vi "Save Acoustic Data.vi"(0 "ID":i32, 1 "base path":path, 5 "Air Temperature":dbl, 7 "Angle":dbl, 9 "Height":dbl, 11 "error in (no error)":errorcluster, 12 "Captured Data":waveform(dbl)) -> (15 "error out":errorcluster)   [LabVIEW 2021]
uses:
  <vilib>/Utility/file.llb/Write Delimited Spreadsheet (DBL).vi
  <vilib>/Utility/file.llb/Write Delimited Spreadsheet (string).vi
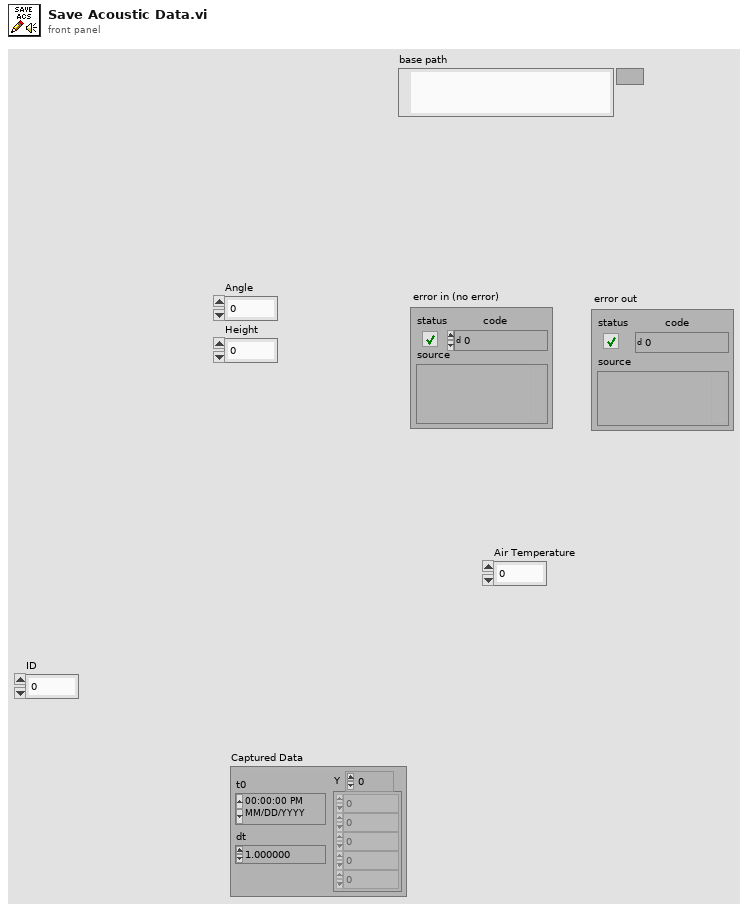
[diagram p1: front panel]
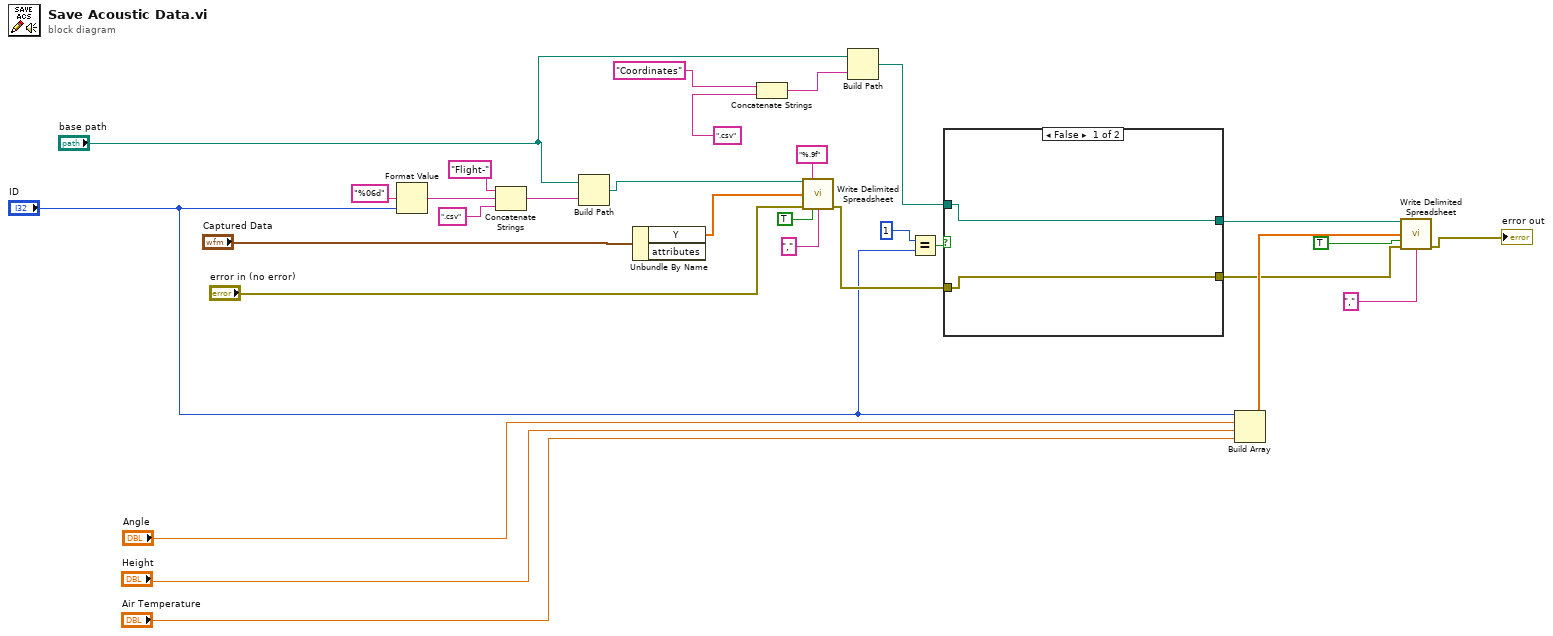
[diagram p0: block diagram]
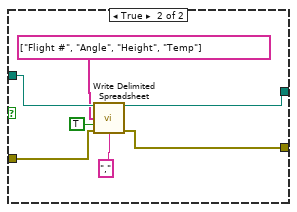
[diagram p2: hidden frame]
diagram:
  n1 = Format Value(format string="%06d", value (0)="ID") -> (output string=w25:string)  [unwired: 1 in]
  n2 = Concatenate Strings("Flight-" ("string"), w25, ".csv") -> (w28:string)
  n3 = Build Path(base path="base path", name or relative path=w28) -> (appended path=w22:path)
  n4 = Unbundle By Name("Captured Data") -> ("Y"=w23:dbl[])  [unwired: 1 out]
  n5 = Concatenate Strings("Coordinates" ("string"), ".csv") -> (w17:string)
  n6 = call-poly <vilib>:"Write Delimited Spreadsheet.vi"("file path (dialog if empty)"=w22, "format (%.3f)"="%.9f" ("format string"), "1D data"=w23, "error in (no error)"="error in (no error)", "transpose? (no:F)"=TRUE, "delimiter (\\t)"="," ("delimiter (Tab)")) -> ("error out"=w4:errorcluster)  [unwired: 8 in, 1 out]
  n7 = Build Path(base path="base path", name or relative path=w17) -> (appended path=w10:path)
  n8 = Equal?(x=1 ("y"), y="ID") -> (x = y?=w11:bool)
  n9 = case shown="False" w11 {
    tunnel: w10 -> [w32 w39]
    tunnel: [w32 w35] -> w6
    tunnel: w4 -> [w31 w34]
    tunnel: [w31 w33] -> w3
    frame False {
    }
    frame True {
      n10 = call-poly <vilib>:"Write Delimited Spreadsheet.vi"("file path (dialog if empty)"=w39, "1D data"=string[] ["Flight #", "Angle", "Height", "Temp"], "append to file? (new file:F)"=TRUE, "error in (no error)"=w34, "delimiter (\\t)"="," ("delimiter (\\t)")) -> ("new file path (Not A Path if cancelled)"=w35:path, "error out"=w33:errorcluster)  [unwired: 9 in]
    }
  }
  n11 = Build Array("ID", "Angle", "Height", "Air Temperature") -> (w15:dbl[])
  n12 = call-poly <vilib>:"Write Delimited Spreadsheet.vi"("file path (dialog if empty)"=w6, "1D data"=w15, "append to file? (new file:F)"=TRUE, "error in (no error)"=w3, "delimiter (\\t)"="," ("delimiter (\\t)")) -> ("error out"=→"error out":errorcluster)  [unwired: 9 in, 1 out]
